vi "Write Reference.vi"(8 "error in (no error)":errorcluster, 10 "Reference":refnum<vi>, 11 "LV Doc in":refnum<class "LV Doc.lvclass">) -> (0 "error out":errorcluster, 3 "LV Doc out":refnum<class "LV Doc.lvclass">)   [LabVIEW 2016, in "LV Doc.lvclass"]
uses:
  LV Doc.lvclass
  LV Doc.lvclass/LV Doc.ctl
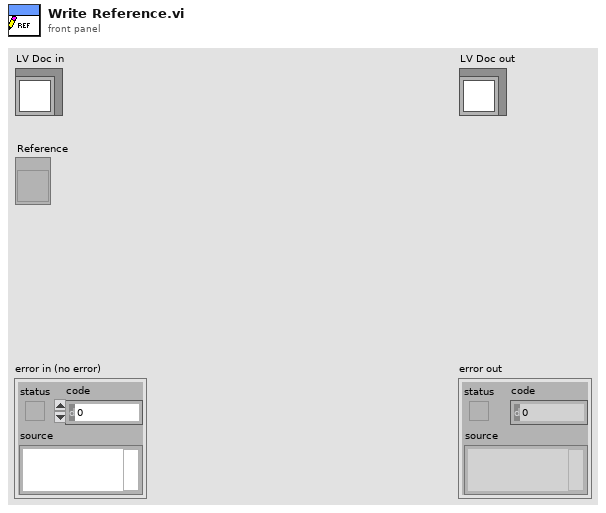
[diagram p1: front panel]
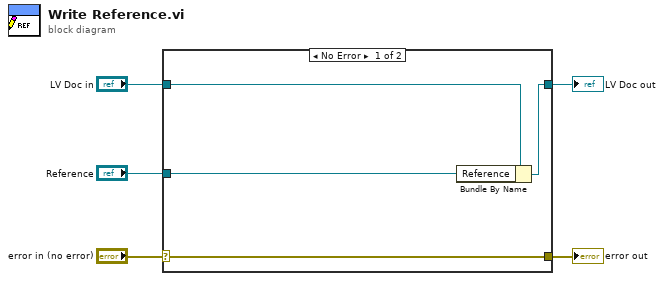
[diagram p0: block diagram]
diagram:
  n1 = case shown="No Error" "error in (no error)" {
    selector: "error in (no error)" -> [w9 w10]
    tunnel: [w9 w10] -> w4
    tunnel: [w7 w11] -> w2
    tunnel: "LV Doc in" -> [w8 w11]
    tunnel: "Reference" -> [w6 _]
    frame No Error {
      n2 = Bundle By Name(cluster=w8, "Reference"=w6) -> (w7:refnum<class "LV Doc.lvclass">)
    }
    frame Error {
    }
  }
  "error out" <- w4
  "LV Doc out" <- w2
